vi "Control VI.vi"() -> ()   [LabVIEW 2018]
uses:
  <vilib>/Instr/_visa.llb/VISA Configure Serial Port (Instr).vi
panel:
  out "Delimitador":string
  out "Baudrate":u32
  out "TetaS":i32
  out "TetaZ":i32
  out "TetaY":i32
  out "TetaX":i32
  in  "Gráficos":bool
  in  "AYUDA":bool
  out "TX DATA":string
  out "RX DATA":string
  in  "MODO DE OPERACIÓN":bool
  in  "Stop":bool
  out "Auto":bool
  out "Manual":bool
  out "Posición Z:":string
  out "Posición Y:":string
  out "Posición X:":string
  in  "SUJETADOR":i32(knob) scale=0.0..50.0
  in  "ACTUADOR Z":i32(knob) scale=0.0..180.0
  in  "ACTUADOR Y":i32(knob) scale=0.0..180.0
  in  "ACTUADOR X":i32(knob) scale=0.0..180.0
  in  "PUERTO DE COMUNICACIÓN":refnum<visa-resource-name>
  # "UNIVERSIDAD DE GUANAJUATO"
  # "DIVISIÓN DE INGENIERÍAS"
  # "RX/TX DATOS"
  # "Manual"
  # "ESTADO DEL MANIPULADOR"
  # "Auto"
  # "CONTROL"
  # "PUERTO COM"
  # "DESCONEXIÓN"
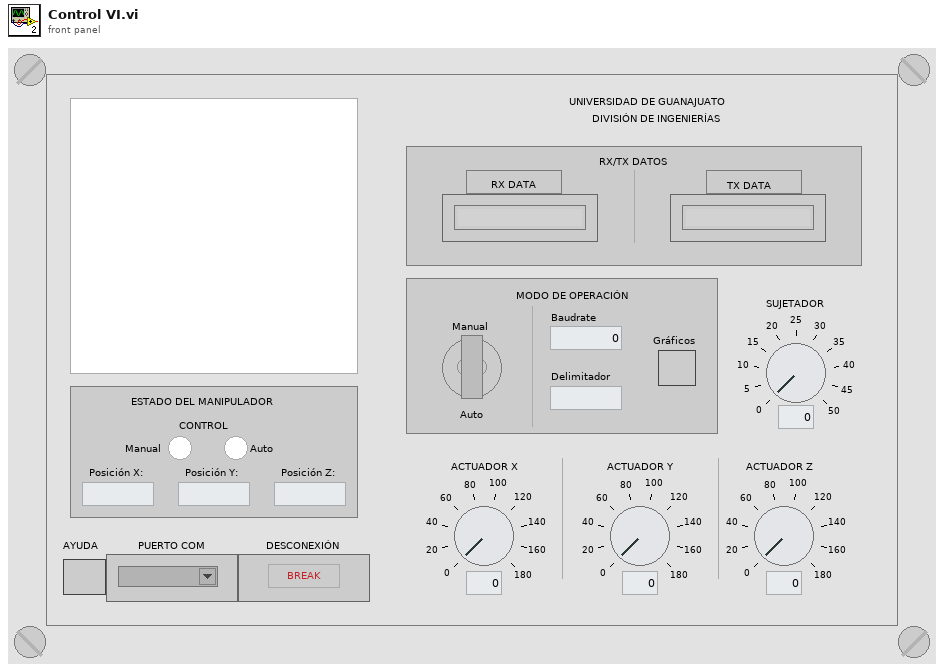
[diagram p1: front panel]
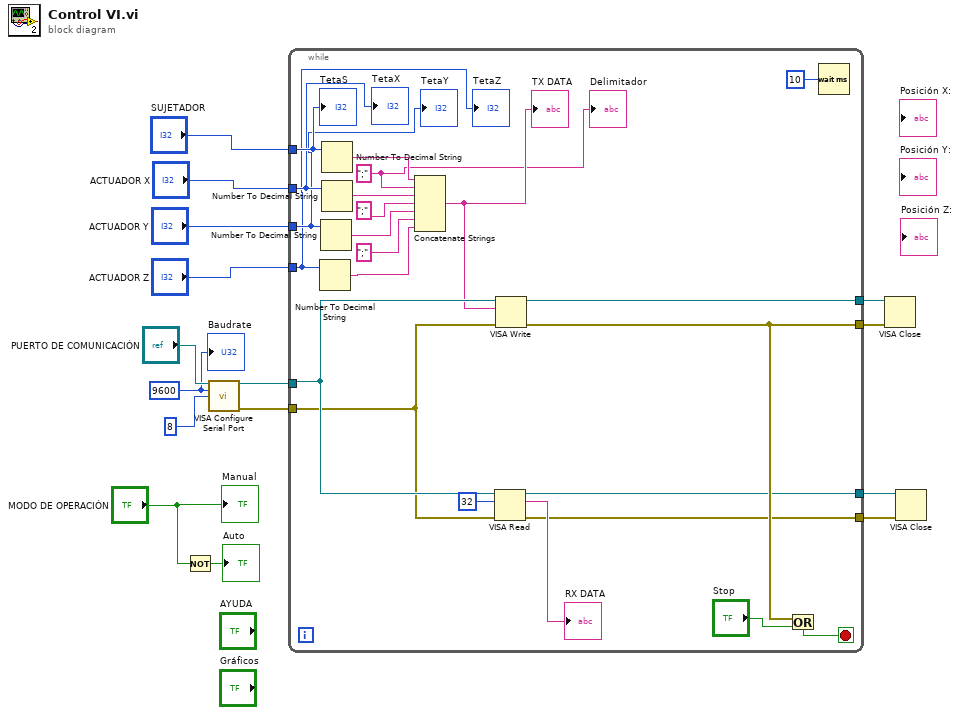
[diagram p0: block diagram]
diagram:
  w1 = u32 9600 ("baud rate (9600)")
  n1 = Not(x="MODO DE OPERACIÓN") -> (.not. x?=→"Auto":bool)
  n2 = call-poly "VISA Configure Serial Port"("VISA resource name"="PUERTO DE COMUNICACIÓN", "baud rate (9600)"=w1, "data bits (8)"=u16 8) -> ("VISA resource name out"=w11:refnum<visa-resource-name>, "error out"=w6:errorcluster)  [unwired: 11 in]
  n3 = while {
    tunnel: w11 -> [w37]
    tunnel: "SUJETADOR" -> [w36]
    tunnel: "ACTUADOR X" -> [w35]
    tunnel: "ACTUADOR Y" -> [w34]
    tunnel: "ACTUADOR Z" -> [w33]
    tunnel: w6 -> [w20]
    tunnel: [w24] -> w5
    tunnel: [w21] -> w4
    tunnel: [w19] -> w3
    tunnel: [w17] -> w2
    stop <- w23 stop-if-true
    w16 = ";" ("string")
    n4 = Number To Decimal String(number=w33) -> (decimal integer string=w27:string)  [unwired: 1 in]
    n5 = Number To Decimal String(number=w34) -> (decimal integer string=w29:string)  [unwired: 1 in]
    n6 = Number To Decimal String(number=w36) -> (decimal integer string=w32:string)  [unwired: 1 in]
    n7 = Number To Decimal String(number=w35) -> (decimal integer string=w31:string)  [unwired: 1 in]
    n8 = Concatenate Strings(w32, w16, w31, ";" ("string"), w29, ";" ("string"), w27) -> (w25:string)
    "TX DATA" <- w25
    n9 = VISA Read(VISA resource name=w37, byte count=u32 32, error in (no error)=w20) -> (VISA resource name out=w19:refnum<visa-resource-name>, read buffer=→"RX DATA":string, error out=w17:errorcluster)  [unwired: 1 out]
    n10 = VISA Write(VISA resource name=w37, write buffer=w25, error in (no error)=w20) -> (VISA resource name out=w24:refnum<visa-resource-name>, error out=w21:errorcluster)  [unwired: 1 out]
    n11 = Or(x=w21, y="Stop") -> (x .or. y?=w23:bool)
    n12 = Wait (ms)(milliseconds to wait=u32 10) -> ()  [unwired: 1 out]
    "TetaS" <- w36
    "TetaX" <- w35
    "TetaY" <- w34
    "TetaZ" <- w33
    "Delimitador" <- w16
  }
  n13 = VISA Close(VISA resource name=w5, error in (no error)=w4) -> ()  [unwired: 1 out]
  n14 = VISA Close(VISA resource name=w3, error in (no error)=w2) -> ()  [unwired: 1 out]
  "Manual" <- "MODO DE OPERACIÓN"
  "Baudrate" <- w1
